vi "Create.vi"(8 "error in (no error)":errorcluster) -> (0 "error out":errorcluster, 3 "GW-SpitOut-Cmd out":refnum<class "GW-SpitOut-Cmd.lvclass">)   [LabVIEW 2013, in "GW-SpitOut-Cmd.lvclass"]
uses:
  GW-SpitOut-Cmd.lvclass
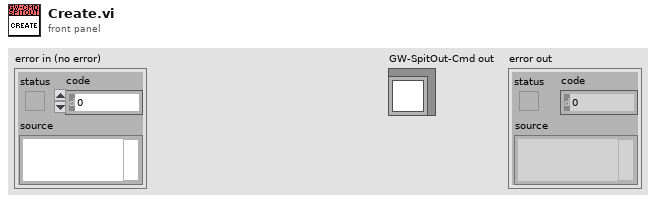
[diagram p1: front panel]
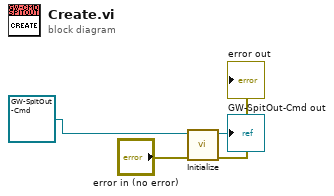
[diagram p0: block diagram]
diagram:
  n1 = call-dynamic "Initialize.vi"("error in (no error)"="error in (no error)", "GW-SpitOut-Cmd in"=refnum<class "GW-SpitOut-Cmd.lvclass"> refnum ("GW-SpitOut-Cmd.lvclass")) -> ("error out"=→"error out":errorcluster, "GW-SpitOut-Cmd out"=→"GW-SpitOut-Cmd out":refnum<class "GW-SpitOut-Cmd.lvclass">)  [unwired: 8 in]
